vi "Size.vi"(8 "error in (no error)":errorcluster, 11 "Enum Array in":refnum<class "Enum Array.lvclass">) -> (0 "error out":errorcluster, 2 "Size":i32, 3 "Enum Array out":refnum<class "Enum Array.lvclass">)   [LabVIEW 2020, in "Data.lvlib" / "Enum Array.lvclass"]
doc: "Return the size of the generic data element."
uses:
  Enum Array.lvclass
  Enum Array.lvclass/Enum Array.ctl
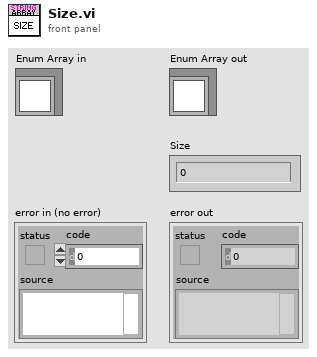
[diagram p1: front panel]
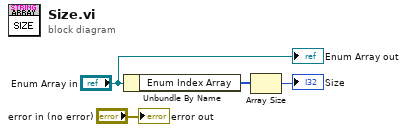
[diagram p0: block diagram]
diagram:
  n1 = Unbundle By Name("Enum Array in") -> ("Enum Index Array"=w1:u32[])
  n2 = Array Size(array=w1) -> (size(s)=→"Size":i32)
  "error out" <- "error in (no error)"
  "Enum Array out" <- "Enum Array in"
